vi "VISA.vi"(8 "error in (no error)":errorcluster, 11 "Cobolt in":refnum<class "Cobolt.lvclass">) -> (0 "error out":errorcluster, 3 "Cobolt out":refnum<class "Cobolt.lvclass">)   [LabVIEW 2012, in "Cobolt.lvclass"]
uses:
  Cobolt.lvclass
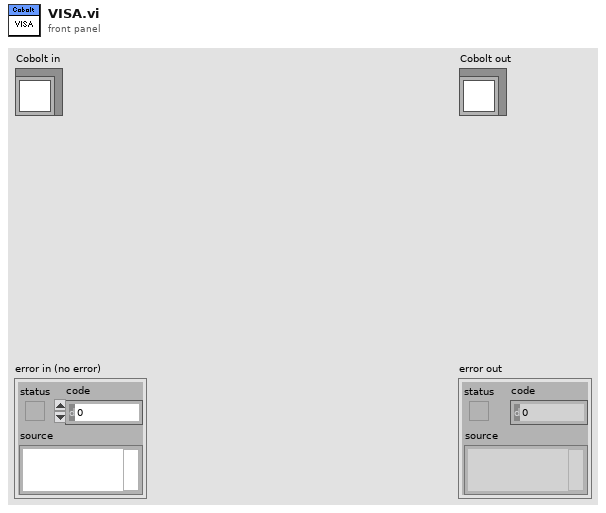
[diagram p1: front panel]
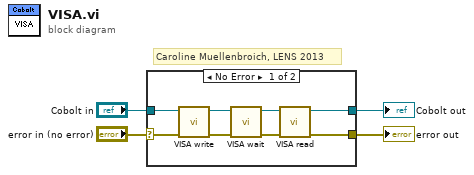
[diagram p0: block diagram]
diagram:
  # "Caroline Muellenbroich, LENS 2013"
  n1 = case shown="No Error" "error in (no error)" {
    selector: "error in (no error)" -> [w8 w14]
    tunnel: [w5 w14] -> w3
    tunnel: [w9 w13] -> w1
    tunnel: "Cobolt in" -> [w12 w13]
    frame No Error {
      n2 = call-dynamic "VISA write.vi"("error in (no error)"=w8, "Cobolt in"=w12) -> ("error out"=w7:errorcluster, "Cobolt out"=w11:refnum<class "Cobolt.lvclass">)  [unwired: 8 in]
      n3 = call-dynamic "VISA wait.vi"("error in (no error)"=w7, "Cobolt in"=w11) -> ("error out"=w6:errorcluster, "Cobolt out"=w10:refnum<class "Cobolt.lvclass">)  [unwired: 8 in]
      n4 = call-dynamic "VISA read.vi"("error in (no error)"=w6, "Cobolt in"=w10) -> ("error out"=w5:errorcluster, "Cobolt out"=w9:refnum<class "Cobolt.lvclass">)  [unwired: 7 in, 1 out]
    }
    frame Error {
    }
  }
  "error out" <- w3
  "Cobolt out" <- w1
